vi "RTS MX5 Data.vi"(4 "Measurement Values in":dbl[][](array[numeric]), 6 "Debug":bool, 8 "Error In":errorcluster, 9 "Measurement Date Times":T1(array[cluster]), 10 "Chamber 1 Data in in":T4 {"Room PID Settings"."Room Dehumid Temperature I (*RM Dehum I1)" max=30000 step=1; "Room PID Settings"."Room Dehumid Temperature P (*RM Dehum P1)" max=30000 step=1; "Room PID Settings"."Room Cool Temperature I (*RM Cool I1)" max=30000 step=1; "Room PID Settings"."Room Cool Temperature P (*RM Cool P1)" max=30000 step=1; "Room PID Settings"."Room Heat I (*RM Heat I1)" max=30000 step=1; "Room PID Settings"."Room Heat P (*RM Heat P1)" max=30000 step=1; "Room PID Settings"."Room Humidity I (*RM Hum I1)" max=30000 step=1; "Room PID Settings"."Room Humidity P (*RM Hum P1)" max=30000 step=1; "Room PID Settings"."Room Dry I (*RM Dry I1)" max=30000 step=1; "Room PID Settings"."Room Dry P(*RM Dry P1)" max=30000 step=1; "Station 8"."Voltage (V):Element 1 Avg" format="%.3g"; "Station 8"."Voltage (V):Element 2 Avg" format="%.3g"; "Station 8"."Max Watt Hours" format="%.3g"; "Station 8"."Power Factor:Element 2" format="%.3g"; "Station 8"."Power Factor:Element 1" format="%.3g"; "Station 8"."Apparent Power (VA):Element 2" format="%.3g"; "Station 8"."Apparent Power (VA):Element 1" format="%.3g"; "Station 8"."Frequency (Hz):Element 1" format="%.3g"; "Station 8"."Time:Element 1" format="%.3g"; "Station 8"."Voltage Crest Factor:Element 2" format="%.3g"; "Station 8"."Voltage Crest Factor:Element 1" format="%.3g"; "Station 8"."Voltage Harmonic (%):Element 2" format="%.3g"; "Station 8"."Voltage Harmonic (%):Element 1" format="%.3g"; "Station 8"."Current Crest Factor:Element 2" format="%.3g"; "Station 8"."Current Crest Factor:Element 1" format="%.3g"; "Station 8"."Voltage (V):Element 1" format="%.3g"; "Station 8"."Voltage (V):Element 2" format="%.3g"; "Station 8"."Watt Hours (Wh):Sigma" format="%.3f"; "Station 8"."Power (W):Sigma" format="%.3g"; "Station 8"."Current (A):Element 2" format="%.3g"; "Station 8"."Current (A):Element 1" format="%.3g"; "Station 7"."Voltage (V):Element 1 Avg" format="%.3g"; "Station 7"."Voltage (V):Element 2 Avg" format="%.3g"; "Station 7"."Max Watt Hours" format="%.3g"; "Station 7"."Power Factor:Element 2" format="%.3g"; "Station 7"."Power Factor:Element 1" format="%.3g"; "Station 7"."Apparent Power (VA):Element 2" format="%.3g"; "Station 7"."Apparent Power (VA):Element 1" format="%.3g"; "Station 7"."Frequency (Hz):Element 1" format="%.3g"; "Station 7"."Time:Element 1" format="%.3g"; "Station 7"."Voltage Crest Factor:Element 2" format="%.3g"; "Station 7"."Voltage Crest Factor:Element 1" format="%.3g"; "Station 7"."Voltage Harmonic (%):Element 2" format="%.3g"; "Station 7"."Voltage Harmonic (%):Element 1" format="%.3g"; "Station 7"."Current Crest Factor:Element 2" format="%.3g"; "Station 7"."Current Crest Factor:Element 1" format="%.3g"; "Station 7"."Voltage (V):Element 1" format="%.3g"; "Station 7"."Voltage (V):Element 2" format="%.3g"; "Station 7"."Watt Hours (Wh):Sigma" format="%.3f"; "Station 7"."Power (W):Sigma" format="%.3g"; "Station 7"."Current (A):Element 2" format="%.3g"; "Station 7"."Current (A):Element 1" format="%.3g"; "Station 6"."Voltage (V):Element 1 Avg" format="%.3g"; "Station 6"."Voltage (V):Element 2 Avg" format="%.3g"; "Station 6"."Max Watt Hours" format="%.3g"; "Station 6"."Power Factor:Element 2" format="%.3g"; "Station 6"."Power Factor:Element 1" format="%.3g"; "Station 6"."Apparent Power (VA):Element 2" format="%.3g"; "Station 6"."Apparent Power (VA):Element 1" format="%.3g"; "Station 6"."Frequency (Hz):Element 1" format="%.3g"; "Station 6"."Time:Element 1" format="%.3g"; "Station 6"."Voltage Crest Factor:Element 2" format="%.3g"; "Station 6"."Voltage Crest Factor:Element 1" format="%.3g"; "Station 6"."Voltage Harmonic (%):Element 2" format="%.3g"; "Station 6"."Voltage Harmonic (%):Element 1" format="%.3g"; "Station 6"."Current Crest Factor:Element 2" format="%.3g"; "Station 6"."Current Crest Factor:Element 1" format="%.3g"; "Station 6"."Voltage (V):Element 1" format="%.3g"; "Station 6"."Voltage (V):Element 2" format="%.3g"; "Station 6"."Watt Hours (Wh):Sigma" format="%.3f"; "Station 6"."Power (W):Sigma" format="%.3g"; "Station 6"."Current (A):Element 2" format="%.3g"; "Station 6"."Current (A):Element 1" format="%.3g"; "Station 5"."Voltage (V):Element 1 Avg" format="%.3g"; "Station 5"."Voltage (V):Element 2 Avg" format="%.3g"; "Station 5"."Max Watt Hours" format="%.3g"; "Station 5"."Power Factor:Element 2" format="%.3g"; "Station 5"."Power Factor:Element 1" format="%.3g"; "Station 5"."Apparent Power (VA):Element 2" format="%.3g"; "Station 5"."Apparent Power (VA):Element 1" format="%.3g"; "Station 5"."Frequency (Hz):Element 1" format="%.3g"; "Station 5"."Time:Element 1" format="%.3g"; "Station 5"."Voltage Crest Factor:Element 2" format="%.3g"; "Station 5"."Voltage Crest Factor:Element 1" format="%.3g"; "Station 5"."Voltage Harmonic (%):Element 2" format="%.3g"; "Station 5"."Voltage Harmonic (%):Element 1" format="%.3g"; "Station 5"."Current Crest Factor:Element 2" format="%.3g"; "Station 5"."Current Crest Factor:Element 1" format="%.3g"; "Station 5"."Voltage (V):Element 1" format="%.3g"; "Station 5"."Voltage (V):Element 2" format="%.3g"; "Station 5"."Watt Hours (Wh):Sigma" format="%.3f"; "Station 5"."Power (W):Sigma" format="%.3g"; "Station 5"."Current (A):Element 2" format="%.3g"; "Station 5"."Current (A):Element 1" format="%.3g"; "Station 4"."Voltage (V):Element 1 Avg" format="%.3g"; "Station 4"."Voltage (V):Element 2 Avg" format="%.3g"; "Station 4"."Max Watt Hours" format="%.3g"; "Station 4"."Power Factor:Element 2" format="%.3g"; "Station 4"."Power Factor:Element 1" format="%.3g"; "Station 4"."Apparent Power (VA):Element 2" format="%.3g"; "Station 4"."Apparent Power (VA):Element 1" format="%.3g"; "Station 4"."Frequency (Hz):Element 1" format="%.3g"; "Station 4"."Time:Element 1" format="%.3g"; "Station 4"."Voltage Crest Factor:Element 2" format="%.3g"; "Station 4"."Voltage Crest Factor:Element 1" format="%.3g"; "Station 4"."Voltage Harmonic (%):Element 2" format="%.3g"; "Station 4"."Voltage Harmonic (%):Element 1" format="%.3g"; "Station 4"."Current Crest Factor:Element 2" format="%.3g"; "Station 4"."Current Crest Factor:Element 1" format="%.3g"; "Station 4"."Voltage (V):Element 1" format="%.3g"; "Station 4"."Voltage (V):Element 2" format="%.3g"; "Station 4"."Watt Hours (Wh):Sigma" format="%.3f"; "Station 4"."Power (W):Sigma" format="%.3g"; "Station 4"."Current (A):Element 2" format="%.3g"; "Station 4"."Current (A):Element 1" format="%.3g"; "Station 3"."Voltage (V):Element 1 Avg" format="%.3g"; "Station 3"."Voltage (V):Element 2 Avg" format="%.3g"; "Station 3"."Max Watt Hours" format="%.3g"; "Station 3"."Power Factor:Element 2" format="%.3g"; "Station 3"."Power Factor:Element 1" format="%.3g"; "Station 3"."Apparent Power (VA):Element 2" format="%.3g"; "Station 3"."Apparent Power (VA):Element 1" format="%.3g"; "Station 3"."Frequency (Hz):Element 1" format="%.3g"; "Station 3"."Time:Element 1" format="%.3g"; "Station 3"."Voltage Crest Factor:Element 2" format="%.3g"; "Station 3"."Voltage Crest Factor:Element 1" format="%.3g"; "Station 3"."Voltage Harmonic (%):Element 2" format="%.3g"; "Station 3"."Voltage Harmonic (%):Element 1" format="%.3g"; "Station 3"."Current Crest Factor:Element 2" format="%.3g"; "Station 3"."Current Crest Factor:Element 1" format="%.3g"; "Station 3"."Voltage (V):Element 1" format="%.3g"; "Station 3"."Voltage (V):Element 2" format="%.3g"; "Station 3"."Watt Hours (Wh):Sigma" format="%.3f"; "Station 3"."Power (W):Sigma" format="%.3g"; "Station 3"."Current (A):Element 2" format="%.3g"; "Station 3"."Current (A):Element 1" format="%.3g"; "Station 2"."Voltage (V):Element 1 Avg" format="%.3g"; "Station 2"."Voltage (V):Element 2 Avg" format="%.3g"; "Station 2"."Max Watt Hours" format="%.3g"; "Station 2"."Power Factor:Element 2" format="%.3g"; "Station 2"."Power Factor:Element 1" format="%.3g"; "Station 2"."Apparent Power (VA):Element 2" format="%.3g"; "Station 2"."Apparent Power (VA):Element 1" format="%.3g"; "Station 2"."Frequency (Hz):Element 1" format="%.3g"; "Station 2"."Time:Element 1" format="%.3g"; "Station 2"."Voltage Crest Factor:Element 2" format="%.3g"; "Station 2"."Voltage Crest Factor:Element 1" format="%.3g"; "Station 2"."Voltage Harmonic (%):Element 2" format="%.3g"; "Station 2"."Voltage Harmonic (%):Element 1" format="%.3g"; "Station 2"."Current Crest Factor:Element 2" format="%.3g"; "Station 2"."Current Crest Factor:Element 1" format="%.3g"; "Station 2"."Voltage (V):Element 1" format="%.3g"; "Station 2"."Voltage (V):Element 2" format="%.3g"; "Station 2"."Watt Hours (Wh):Sigma" format="%.3f"; "Station 2"."Power (W):Sigma" format="%.3g"; "Station 2"."Current (A):Element 2" format="%.3g"; "Station 2"."Current (A):Element 1" format="%.3g"; "Station 1"."Voltage (V):Element 1 Avg" format="%.3g"; "Station 1"."Voltage (V):Element 2 Avg" format="%.3g"; "Station 1"."Max Watt Hours" format="%.3g"; "Station 1"."Power Factor:Element 2" format="%.3g"; "Station 1"."Power Factor:Element 1" format="%.3g"; "Station 1"."Apparent Power (VA):Element 2" format="%.3g"; "Station 1"."Apparent Power (VA):Element 1" format="%.3g"; "Station 1"."Frequency (Hz):Element 1" format="%.3g"; "Station 1"."Time:Element 1" format="%.3g"; "Station 1"."Voltage Crest Factor:Element 2" format="%.3g"; "Station 1"."Voltage Crest Factor:Element 1" format="%.3g"; "Station 1"."Voltage Harmonic (%):Element 2" format="%.3g"; "Station 1"."Voltage Harmonic (%):Element 1" format="%.3g"; "Station 1"."Current Crest Factor:Element 2" format="%.3g"; "Station 1"."Current Crest Factor:Element 1" format="%.3g"; "Station 1"."Voltage (V):Element 1" format="%.3g"; "Station 1"."Voltage (V):Element 2" format="%.3g"; "Station 1"."Watt Hours (Wh):Sigma" format="%.3f"; "Station 1"."Power (W):Sigma" format="%.3g"; "Station 1"."Current (A):Element 2" format="%.3g"; "Station 1"."Current (A):Element 1" format="%.3g"}, 11 "MX":T2={"Base Time"=0, "Session Number"=0, "Last Data Number"={"High"=-1, "Low"=4294967295}, "Channel List"=[], "FIFO Number (0)"=0, "Channel Number (1)"=1, "Select FIFO or Channel (F:Channel)"=FALSE, "MX100 Data"={"Measurement Values out"=[], "Date/Time"=""}} {"Channel Number (1)" min=1 max=60 step=1; "FIFO Number (0)" min=-1 max=2 step=1}) -> (0 "Error Out":errorcluster, 2 "Chamber 1 Data out":T4 {"Room PID Settings"."Room Dehumid Temperature I (*RM Dehum I1)" max=30000 step=1; "Room PID Settings"."Room Dehumid Temperature P (*RM Dehum P1)" max=30000 step=1; "Room PID Settings"."Room Cool Temperature I (*RM Cool I1)" max=30000 step=1; "Room PID Settings"."Room Cool Temperature P (*RM Cool P1)" max=30000 step=1; "Room PID Settings"."Room Heat I (*RM Heat I1)" max=30000 step=1; "Room PID Settings"."Room Heat P (*RM Heat P1)" max=30000 step=1; "Room PID Settings"."Room Humidity I (*RM Hum I1)" max=30000 step=1; "Room PID Settings"."Room Humidity P (*RM Hum P1)" max=30000 step=1; "Room PID Settings"."Room Dry I (*RM Dry I1)" max=30000 step=1; "Room PID Settings"."Room Dry P(*RM Dry P1)" max=30000 step=1; "Station 8"."Voltage (V):Element 1 Avg" format="%.3g"; "Station 8"."Voltage (V):Element 2 Avg" format="%.3g"; "Station 8"."Max Watt Hours" format="%.3g"; "Station 8"."Power Factor:Element 2" format="%.3g"; "Station 8"."Power Factor:Element 1" format="%.3g"; "Station 8"."Apparent Power (VA):Element 2" format="%.3g"; "Station 8"."Apparent Power (VA):Element 1" format="%.3g"; "Station 8"."Frequency (Hz):Element 1" format="%.3g"; "Station 8"."Time:Element 1" format="%.3g"; "Station 8"."Voltage Crest Factor:Element 2" format="%.3g"; "Station 8"."Voltage Crest Factor:Element 1" format="%.3g"; "Station 8"."Voltage Harmonic (%):Element 2" format="%.3g"; "Station 8"."Voltage Harmonic (%):Element 1" format="%.3g"; "Station 8"."Current Crest Factor:Element 2" format="%.3g"; "Station 8"."Current Crest Factor:Element 1" format="%.3g"; "Station 8"."Voltage (V):Element 1" format="%.3g"; "Station 8"."Voltage (V):Element 2" format="%.3g"; "Station 8"."Watt Hours (Wh):Sigma" format="%.3f"; "Station 8"."Power (W):Sigma" format="%.3g"; "Station 8"."Current (A):Element 2" format="%.3g"; "Station 8"."Current (A):Element 1" format="%.3g"; "Station 7"."Voltage (V):Element 1 Avg" format="%.3g"; "Station 7"."Voltage (V):Element 2 Avg" format="%.3g"; "Station 7"."Max Watt Hours" format="%.3g"; "Station 7"."Power Factor:Element 2" format="%.3g"; "Station 7"."Power Factor:Element 1" format="%.3g"; "Station 7"."Apparent Power (VA):Element 2" format="%.3g"; "Station 7"."Apparent Power (VA):Element 1" format="%.3g"; "Station 7"."Frequency (Hz):Element 1" format="%.3g"; "Station 7"."Time:Element 1" format="%.3g"; "Station 7"."Voltage Crest Factor:Element 2" format="%.3g"; "Station 7"."Voltage Crest Factor:Element 1" format="%.3g"; "Station 7"."Voltage Harmonic (%):Element 2" format="%.3g"; "Station 7"."Voltage Harmonic (%):Element 1" format="%.3g"; "Station 7"."Current Crest Factor:Element 2" format="%.3g"; "Station 7"."Current Crest Factor:Element 1" format="%.3g"; "Station 7"."Voltage (V):Element 1" format="%.3g"; "Station 7"."Voltage (V):Element 2" format="%.3g"; "Station 7"."Watt Hours (Wh):Sigma" format="%.3f"; "Station 7"."Power (W):Sigma" format="%.3g"; "Station 7"."Current (A):Element 2" format="%.3g"; "Station 7"."Current (A):Element 1" format="%.3g"; "Station 6"."Voltage (V):Element 1 Avg" format="%.3g"; "Station 6"."Voltage (V):Element 2 Avg" format="%.3g"; "Station 6"."Max Watt Hours" format="%.3g"; "Station 6"."Power Factor:Element 2" format="%.3g"; "Station 6"."Power Factor:Element 1" format="%.3g"; "Station 6"."Apparent Power (VA):Element 2" format="%.3g"; "Station 6"."Apparent Power (VA):Element 1" format="%.3g"; "Station 6"."Frequency (Hz):Element 1" format="%.3g"; "Station 6"."Time:Element 1" format="%.3g"; "Station 6"."Voltage Crest Factor:Element 2" format="%.3g"; "Station 6"."Voltage Crest Factor:Element 1" format="%.3g"; "Station 6"."Voltage Harmonic (%):Element 2" format="%.3g"; "Station 6"."Voltage Harmonic (%):Element 1" format="%.3g"; "Station 6"."Current Crest Factor:Element 2" format="%.3g"; "Station 6"."Current Crest Factor:Element 1" format="%.3g"; "Station 6"."Voltage (V):Element 1" format="%.3g"; "Station 6"."Voltage (V):Element 2" format="%.3g"; "Station 6"."Watt Hours (Wh):Sigma" format="%.3f"; "Station 6"."Power (W):Sigma" format="%.3g"; "Station 6"."Current (A):Element 2" format="%.3g"; "Station 6"."Current (A):Element 1" format="%.3g"; "Station 5"."Voltage (V):Element 1 Avg" format="%.3g"; "Station 5"."Voltage (V):Element 2 Avg" format="%.3g"; "Station 5"."Max Watt Hours" format="%.3g"; "Station 5"."Power Factor:Element 2" format="%.3g"; "Station 5"."Power Factor:Element 1" format="%.3g"; "Station 5"."Apparent Power (VA):Element 2" format="%.3g"; "Station 5"."Apparent Power (VA):Element 1" format="%.3g"; "Station 5"."Frequency (Hz):Element 1" format="%.3g"; "Station 5"."Time:Element 1" format="%.3g"; "Station 5"."Voltage Crest Factor:Element 2" format="%.3g"; "Station 5"."Voltage Crest Factor:Element 1" format="%.3g"; "Station 5"."Voltage Harmonic (%):Element 2" format="%.3g"; "Station 5"."Voltage Harmonic (%):Element 1" format="%.3g"; "Station 5"."Current Crest Factor:Element 2" format="%.3g"; "Station 5"."Current Crest Factor:Element 1" format="%.3g"; "Station 5"."Voltage (V):Element 1" format="%.3g"; "Station 5"."Voltage (V):Element 2" format="%.3g"; "Station 5"."Watt Hours (Wh):Sigma" format="%.3f"; "Station 5"."Power (W):Sigma" format="%.3g"; "Station 5"."Current (A):Element 2" format="%.3g"; "Station 5"."Current (A):Element 1" format="%.3g"; "Station 4"."Voltage (V):Element 1 Avg" format="%.3g"; "Station 4"."Voltage (V):Element 2 Avg" format="%.3g"; "Station 4"."Max Watt Hours" format="%.3g"; "Station 4"."Power Factor:Element 2" format="%.3g"; "Station 4"."Power Factor:Element 1" format="%.3g"; "Station 4"."Apparent Power (VA):Element 2" format="%.3g"; "Station 4"."Apparent Power (VA):Element 1" format="%.3g"; "Station 4"."Frequency (Hz):Element 1" format="%.3g"; "Station 4"."Time:Element 1" format="%.3g"; "Station 4"."Voltage Crest Factor:Element 2" format="%.3g"; "Station 4"."Voltage Crest Factor:Element 1" format="%.3g"; "Station 4"."Voltage Harmonic (%):Element 2" format="%.3g"; "Station 4"."Voltage Harmonic (%):Element 1" format="%.3g"; "Station 4"."Current Crest Factor:Element 2" format="%.3g"; "Station 4"."Current Crest Factor:Element 1" format="%.3g"; "Station 4"."Voltage (V):Element 1" format="%.3g"; "Station 4"."Voltage (V):Element 2" format="%.3g"; "Station 4"."Watt Hours (Wh):Sigma" format="%.3f"; "Station 4"."Power (W):Sigma" format="%.3g"; "Station 4"."Current (A):Element 2" format="%.3g"; "Station 4"."Current (A):Element 1" format="%.3g"; "Station 3"."Voltage (V):Element 1 Avg" format="%.3g"; "Station 3"."Voltage (V):Element 2 Avg" format="%.3g"; "Station 3"."Max Watt Hours" format="%.3g"; "Station 3"."Power Factor:Element 2" format="%.3g"; "Station 3"."Power Factor:Element 1" format="%.3g"; "Station 3"."Apparent Power (VA):Element 2" format="%.3g"; "Station 3"."Apparent Power (VA):Element 1" format="%.3g"; "Station 3"."Frequency (Hz):Element 1" format="%.3g"; "Station 3"."Time:Element 1" format="%.3g"; "Station 3"."Voltage Crest Factor:Element 2" format="%.3g"; "Station 3"."Voltage Crest Factor:Element 1" format="%.3g"; "Station 3"."Voltage Harmonic (%):Element 2" format="%.3g"; "Station 3"."Voltage Harmonic (%):Element 1" format="%.3g"; "Station 3"."Current Crest Factor:Element 2" format="%.3g"; "Station 3"."Current Crest Factor:Element 1" format="%.3g"; "Station 3"."Voltage (V):Element 1" format="%.3g"; "Station 3"."Voltage (V):Element 2" format="%.3g"; "Station 3"."Watt Hours (Wh):Sigma" format="%.3f"; "Station 3"."Power (W):Sigma" format="%.3g"; "Station 3"."Current (A):Element 2" format="%.3g"; "Station 3"."Current (A):Element 1" format="%.3g"; "Station 2"."Voltage (V):Element 1 Avg" format="%.3g"; "Station 2"."Voltage (V):Element 2 Avg" format="%.3g"; "Station 2"."Max Watt Hours" format="%.3g"; "Station 2"."Power Factor:Element 2" format="%.3g"; "Station 2"."Power Factor:Element 1" format="%.3g"; "Station 2"."Apparent Power (VA):Element 2" format="%.3g"; "Station 2"."Apparent Power (VA):Element 1" format="%.3g"; "Station 2"."Frequency (Hz):Element 1" format="%.3g"; "Station 2"."Time:Element 1" format="%.3g"; "Station 2"."Voltage Crest Factor:Element 2" format="%.3g"; "Station 2"."Voltage Crest Factor:Element 1" format="%.3g"; "Station 2"."Voltage Harmonic (%):Element 2" format="%.3g"; "Station 2"."Voltage Harmonic (%):Element 1" format="%.3g"; "Station 2"."Current Crest Factor:Element 2" format="%.3g"; "Station 2"."Current Crest Factor:Element 1" format="%.3g"; "Station 2"."Voltage (V):Element 1" format="%.3g"; "Station 2"."Voltage (V):Element 2" format="%.3g"; "Station 2"."Watt Hours (Wh):Sigma" format="%.3f"; "Station 2"."Power (W):Sigma" format="%.3g"; "Station 2"."Current (A):Element 2" format="%.3g"; "Station 2"."Current (A):Element 1" format="%.3g"; "Station 1"."Voltage (V):Element 1 Avg" format="%.3g"; "Station 1"."Voltage (V):Element 2 Avg" format="%.3g"; "Station 1"."Max Watt Hours" format="%.3g"; "Station 1"."Power Factor:Element 2" format="%.3g"; "Station 1"."Power Factor:Element 1" format="%.3g"; "Station 1"."Apparent Power (VA):Element 2" format="%.3g"; "Station 1"."Apparent Power (VA):Element 1" format="%.3g"; "Station 1"."Frequency (Hz):Element 1" format="%.3g"; "Station 1"."Time:Element 1" format="%.3g"; "Station 1"."Voltage Crest Factor:Element 2" format="%.3g"; "Station 1"."Voltage Crest Factor:Element 1" format="%.3g"; "Station 1"."Voltage Harmonic (%):Element 2" format="%.3g"; "Station 1"."Voltage Harmonic (%):Element 1" format="%.3g"; "Station 1"."Current Crest Factor:Element 2" format="%.3g"; "Station 1"."Current Crest Factor:Element 1" format="%.3g"; "Station 1"."Voltage (V):Element 1" format="%.3g"; "Station 1"."Voltage (V):Element 2" format="%.3g"; "Station 1"."Watt Hours (Wh):Sigma" format="%.3f"; "Station 1"."Power (W):Sigma" format="%.3g"; "Station 1"."Current (A):Element 2" format="%.3g"; "Station 1"."Current (A):Element 1" format="%.3g"})   [LabVIEW 2016]
uses:
  Type Definitions/RTS Chamber Data.ctl
  Utility/Type Definitions/UTILITY Power Data.ctl
  Type Definitions/RTS Chamber TCs.ctl
  Type Definitions/RTS MX5 AUX Data.ctl
  Drivers/WAGO 750-881/Type Definitions/Wago Door Relays.ctl
  Drivers/WAGO 750-881/Type Definitions/Wago Contactor Settings.ctl
  Drivers/WAGO 750-881/Type Definitions/Wago Ground Leakage.ctl
  Drivers/WAGO 750-881/Type Definitions/Wago Measured Input Data.ctl
  Drivers/WAGO 750-881/Type Definitions/Wago Room Setpoint Targets.ctl
  Drivers/WAGO 750-881/Type Definitions/Wago Room PID Settings.ctl
  Drivers/WAGO 750-881/Type Definitions/Wago Room Condtions.ctl
  Drivers/Yokogawa MX100/Type Definitions/MX100 Initialization.ctl
  Drivers/Yokogawa MX100/Type Definitions/MX100 Data.ctl
panel:
  # "APLUS"
  # "MX100"
  # "Wago Controller"
  # "APLUS"
  # "MX100"
  # "Wago Controller"
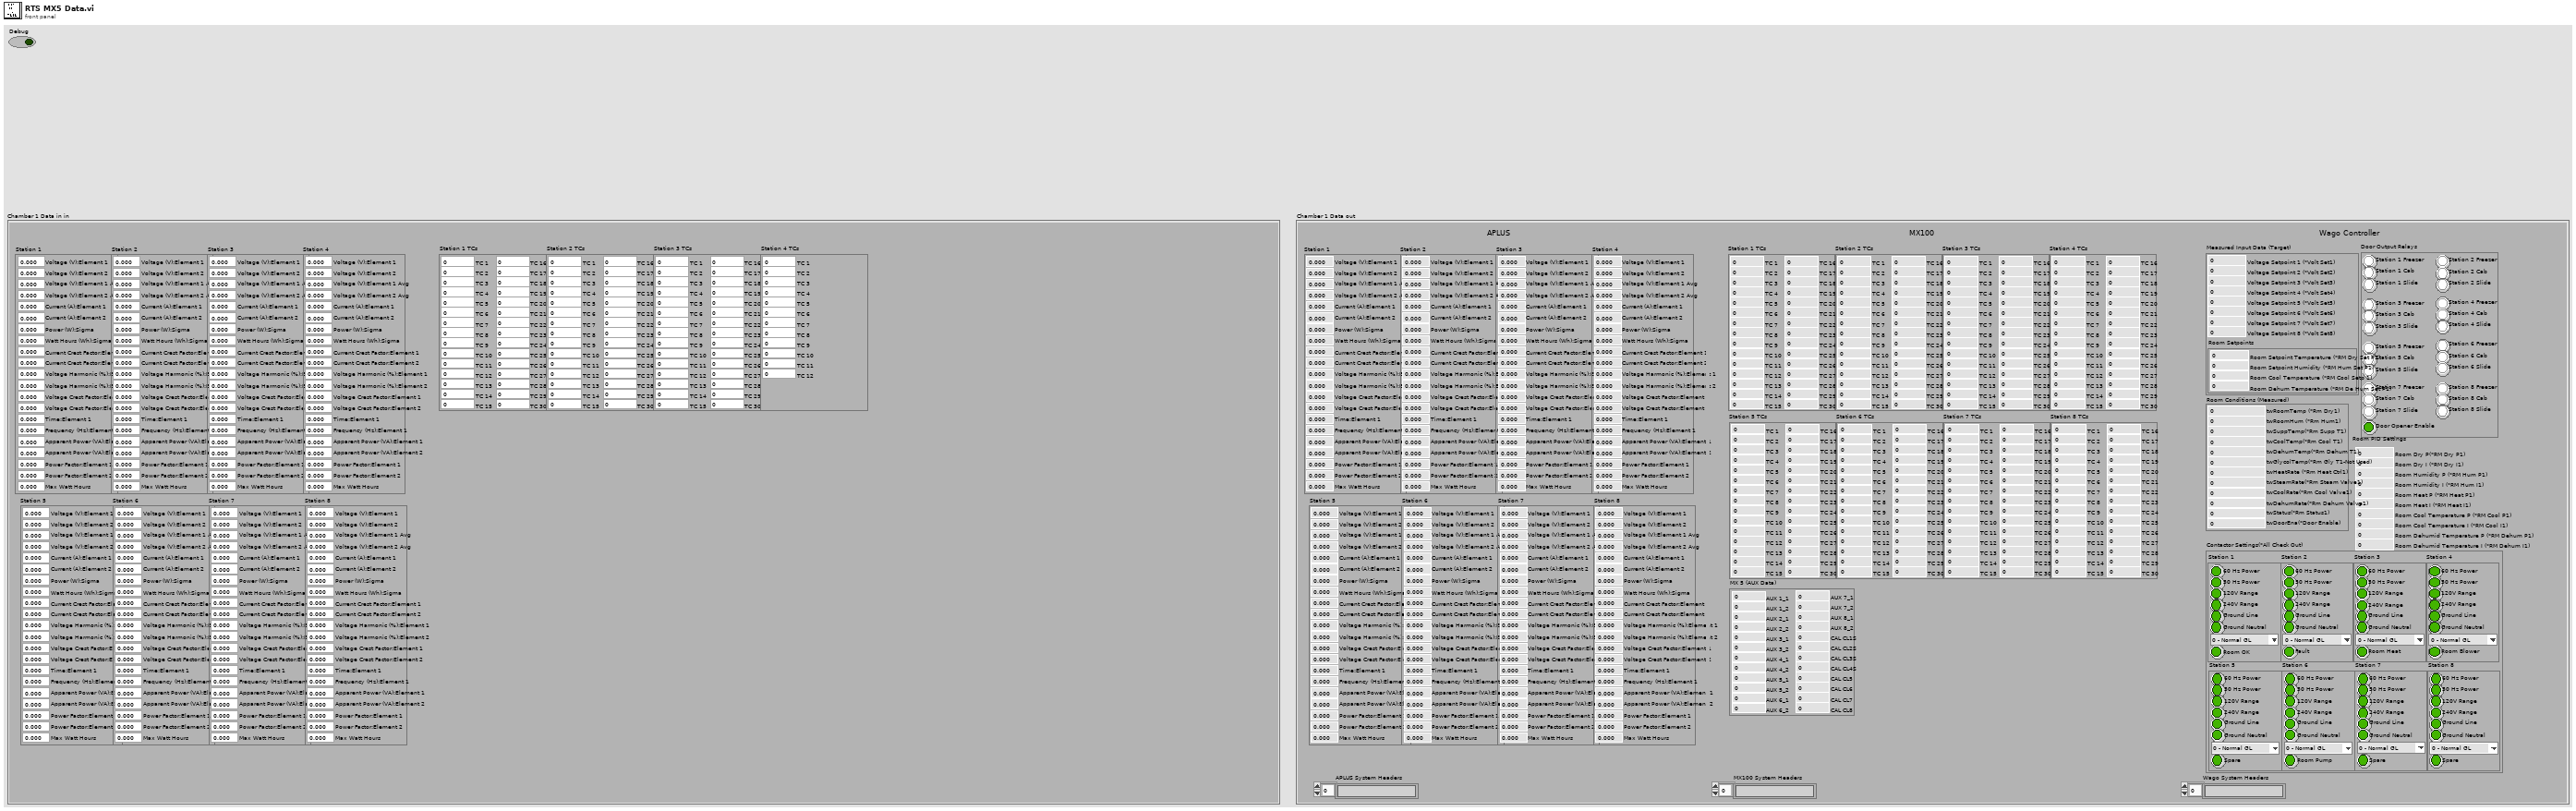
[diagram p1: front panel]
types:
  T1 = cluster{"Measurement Time":u32, "Milli Second":i32}[]
  T2 = typedef "MX100 Initialization.ctl" = cluster{"Base Time":i32, "Session Number":i32, "Last Data Number":cluster{"High":i32, "Low":u32}, "Channel List":string[], "FIFO Number (0)":i32, "Channel Number (1)":i32, "Select FIFO or Channel (F:Channel)":bool, "MX100 Data":T3}
  T3 = typedef "MX100 Data.ctl" = cluster{"Measurement Values out":dbl[], "Date/Time":string}
  T4 = typedef "RTS Chamber Data.ctl" = cluster{"Station 1":T5, "Station 2":T5, "Station 3":T5, "Station 4":T5, "Station 5":T5, "Station 6":T5, "Station 7":T5, "Station 8":T5, "Station 1 TCs":T6, "Station 2 TCs":T6, "Station 3 TCs":T6, "Station 4 TCs":T6, "Station 5 TCs":T6, "Station 6 TCs":T6, "Station 7 TCs":T6, "Station 8 TCs":T6, "MX 5 (AUX Data)":T7, "Door Output Relays":T8, "Contactor Settings(*All Check Out)":T9, "Measured Input Data (Target)":T11, "Room PID Settings":T13, "Room Conditions (Measured)":T14, "APLUS System Headers":string[], "MX100 System Headers":string[], "Wago System Headers":string[]}
  T5 = typedef "UTILITY Power Data.ctl" = cluster{"Current (A):Element 1":dbl, "Current (A):Element 2":dbl, "Power (W):Sigma":dbl, "Watt Hours (Wh):Sigma":dbl, "Voltage (V):Element 2":dbl, "Voltage (V):Element 1":dbl, "Current Crest Factor:Element 1":dbl, "Current Crest Factor:Element 2":dbl, "Voltage Harmonic (%):Element 1":dbl, "Voltage Harmonic (%):Element 2":dbl, "Voltage Crest Factor:Element 1":dbl, "Voltage Crest Factor:Element 2":dbl, "Time:Element 1":dbl, "Frequency (Hz):Element 1":dbl, "Apparent Power (VA):Element 1":dbl, "Apparent Power (VA):Element 2":dbl, "Power Factor:Element 1":dbl, "Power Factor:Element 2":dbl, "Max Watt Hours":dbl, "Voltage (V):Element 2 Avg":dbl, "Voltage (V):Element 1 Avg":dbl}
  T6 = typedef "RTS Chamber TCs.ctl" = cluster{"TC 1":dbl, "TC 2":dbl, "TC 3":dbl, "TC 4":dbl, "TC 5":dbl, "TC 6":dbl, "TC 7":dbl, "TC 8":dbl, "TC 9":dbl, "TC 10":dbl, "TC 11":dbl, "TC 12":dbl, "TC 13":dbl, "TC 14":dbl, "TC 15":dbl, "TC 16":dbl, "TC 17":dbl, "TC 18":dbl, "TC 19":dbl, "TC 20":dbl, "TC 21":dbl, "TC 22":dbl, "TC 23":dbl, "TC 24":dbl, "TC 25":dbl, "TC 26":dbl, "TC 27":dbl, "TC 28":dbl, "TC 29":dbl, "TC 30":dbl}
  T7 = typedef "RTS MX5 AUX Data.ctl" = cluster{"AUX 1_1":dbl, "AUX 1_2":dbl, "AUX 2_1":dbl, "AUX 2_2":dbl, "AUX 3_1":dbl, "AUX 3_2":dbl, "AUX 4_1":dbl, "AUX 4_2":dbl, "AUX 5_1":dbl, "AUX 5_2":dbl, "AUX 6_1":dbl, "AUX 6_2":dbl, "AUX 7_1":dbl, "AUX 7_2":dbl, "AUX 8_1":dbl, "AUX 8_2":dbl, "CAL CL1S":dbl, "CAL CL2S":dbl, "CAL CL3S":dbl, "CAL CL4S":dbl, "CAL CL5":dbl, "CAL CL6":dbl, "CAL CL7":dbl, "CAL CL8":dbl}
  T8 = typedef "Wago Door Relays.ctl" = cluster{"Station 1 Freezer":bool, "Station 1 Cab":bool, "Station 1 Slide":bool, "Station 2 Freezer":bool, "Station 2 Cab":bool, "Station 2 Slide":bool, "Station 3 Freezer":bool, "Station 3 Cab":bool, "Station 3 Slide":bool, "Station 4 Freezer":bool, "Station 4 Cab":bool, "Station 4 Slide":bool, "Station 5 Freezer":bool, "Station 5 Cab":bool, "Station 5 Slide":bool, "Station 6 Freezer":bool, "Station 6 Cab":bool, "Station 6 Slide":bool, "Station 7 Freezer":bool, "Station 7 Cab":bool, "Station 7 Slide":bool, "Station 8 Freezer":bool, "Station 8 Cab":bool, "Station 8 Slide":bool, "Door Opener Enable":bool}
  T9 = typedef "Wago Contactor Settings.ctl" = cluster{"Station 1":cluster{"60 Hz Power":bool, "50 Hz Power":bool, "120V Range":bool, "240V Range":bool, "Ground Line":bool, "Ground Neutral":bool, "Room OK":bool, "Ground Leakage":T10}, "Station 2":cluster{"60 Hz Power":bool, "50 Hz Power":bool, "120V Range":bool, "240V Range":bool, "Ground Line":bool, "Ground Neutral":bool, "Fault":bool, "Ground Leakage":T10}, "Station 3":cluster{"60 Hz Power":bool, "50 Hz Power":bool, "120V Range":bool, "240V Range":bool, "Ground Line":bool, "Ground Neutral":bool, "Room Heat":bool, "Ground Leakage":T10}, "Station 4":cluster{"60 Hz Power":bool, "50 Hz Power":bool, "120V Range":bool, "240V Range":bool, "Ground Line":bool, "Ground Neutral":bool, "Room Blower":bool, "Ground Leakage":T10}, "Station 5":cluster{"60 Hz Power":bool, "50 Hz Power":bool, "120V Range":bool, "240V Range":bool, "Ground Line":bool, "Ground Neutral":bool, "Spare":bool, "Ground Leakage":T10}, "Station 6":cluster{"60 Hz Power":bool, "50 Hz Power":bool, "120V Range":bool, "240V Range":bool, "Ground Line":bool, "Ground Neutral":bool, "Room Pump":bool, "Ground Leakage":T10}, "Station 7":cluster{"60 Hz Power":bool, "50 Hz Power":bool, "120V Range":bool, "240V Range":bool, "Ground Line":bool, "Ground Neutral":bool, "Spare":bool, "Ground Leakage":T10}, "Station 8":cluster{"60 Hz Power":bool, "50 Hz Power":bool, "120V Range":bool, "240V Range":bool, "Ground Line":bool, "Ground Neutral":bool, "Spare":bool, "Ground Leakage":T10}}
  T10 = typedef "Wago Ground Leakage.ctl" = enum16{"0 - Normal GL", "1 - Measure GL"}
  T11 = typedef "Wago Measured Input Data.ctl" = cluster{"Voltage Setpoint 1 (*Volt Set1)":dbl, "Voltage Setpoint 2 (*Volt Set2)":dbl, "Voltage Setpoint 3 (*Volt Set3)":dbl, "Voltage Setpoint 4 (*Volt Set4)":dbl, "Voltage Setpoint 5 (*Volt Set5)":dbl, "Voltage Setpoint 6 (*Volt Set6)":dbl, "Voltage Setpoint 7 (*Volt Set7)":dbl, "Voltage Setpoint 8 (*Volt Set8)":dbl, "Room Setpoints":T12}
  T12 = typedef "Wago Room Setpoint Targets.ctl" = cluster{"Room Setpoint Temperature (*RM Dry Set P1)":dbl, "Room Setpoint Humidity (*RM Hum Set P1)":dbl, "Room Cool Temperature (*RM Cool Setp 1)":dbl, "Room Dehum Temperature (*RM De Hum Set P1)":dbl}
  T13 = typedef "Wago Room PID Settings.ctl" = cluster{"Room Dry P(*RM Dry P1)":u16, "Room Dry I (*RM Dry I1)":u16, "Room Humidity P (*RM Hum P1)":u16, "Room Humidity I (*RM Hum I1)":u16, "Room Heat P (*RM Heat P1)":u16, "Room Heat I (*RM Heat I1)":u16, "Room Cool Temperature P (*RM Cool P1)":u16, "Room Cool Temperature I (*RM Cool I1)":u16, "Room Dehumid Temperature P (*RM Dehum P1)":u16, "Room Dehumid Temperature I (*RM Dehum I1)":u16}
  T14 = typedef "Wago Room Condtions.ctl" = cluster{"twDoorEna(*Door Enable)":u16, "twStatus(*Rm Status1)":u16, "twRoomTemp (*Rm Dry1)":dbl, "twRoomHum (*Rm Hum1)":dbl, "twSuppTemp(*Rm Supp T1)":dbl, "twCoolTemp(*Rm Cool T1)":dbl, "twDehumTemp(*Rm Dehum T1)":dbl, "twGlycolTemp(*Rm Gly T1-Not Used)":dbl, "twDehumRate(*Rm Dehum Valve1)":dbl, "twCoolRate(*Rm Cool Valve1)":dbl, "twSteamRate(*Rm Steam Valve1)":dbl, "twHeatRate (*Rm Heat Ctrl1)":dbl}
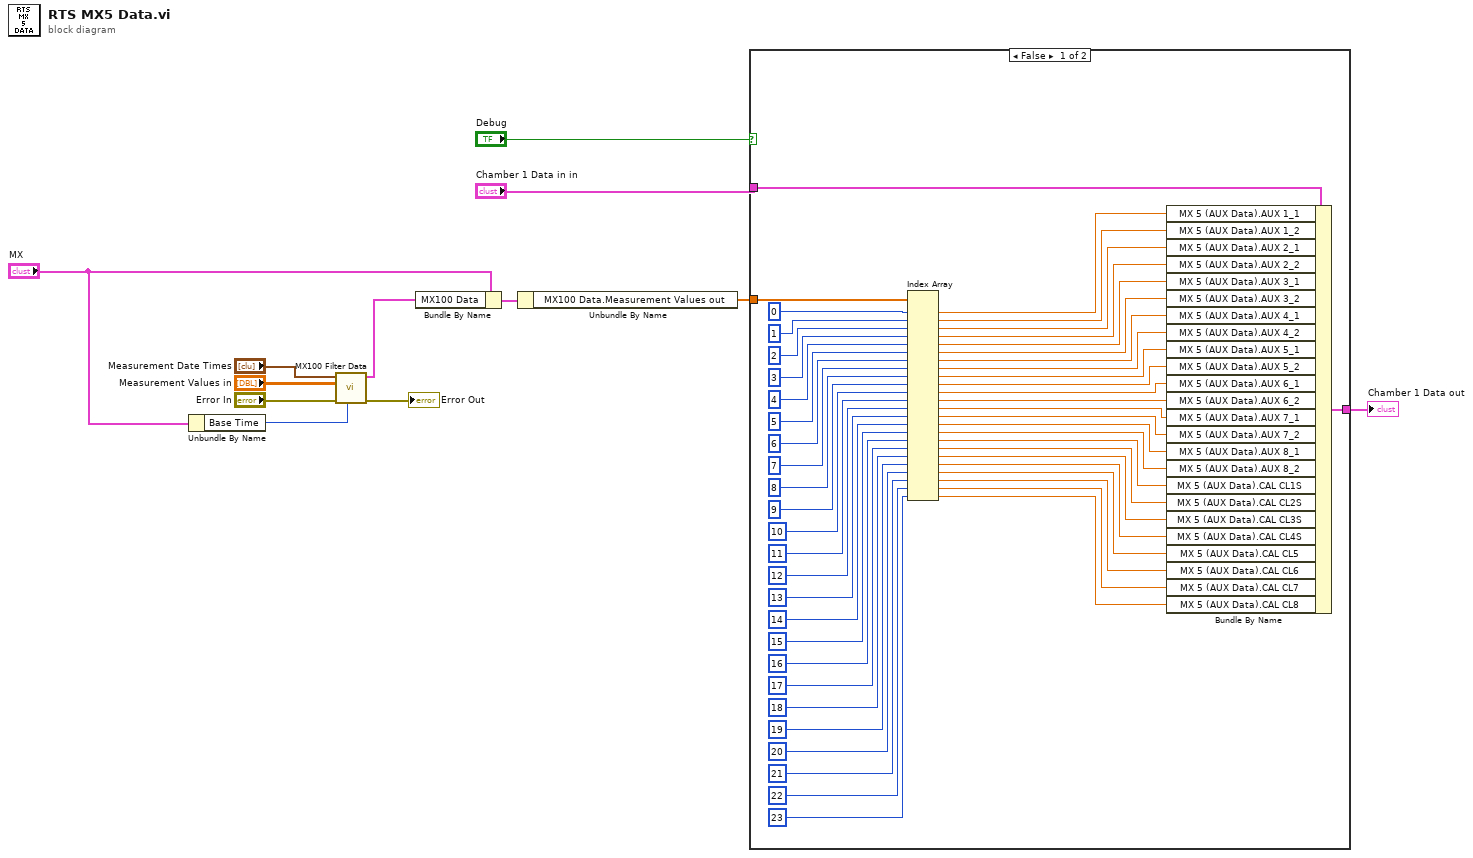
[diagram p0: block diagram]
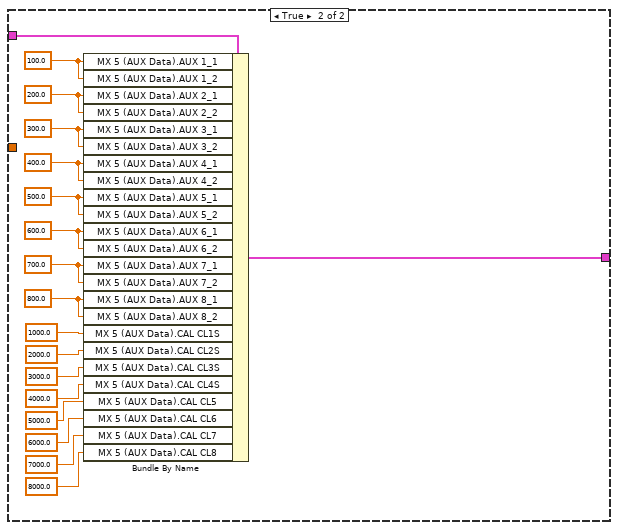
[diagram p2: hidden frame]
diagram:
  n1 = Unbundle By Name("MX") -> ("Base Time"=w8:i32)
  n2 = call "MX100 Filter Data.vi"("Base Time"=w8, "error in (no error)"="Error In", "Measurement Values in"="Measurement Values in", "Measurement Date Times"="Measurement Date Times") -> ("error out"=→"Error Out":errorcluster, "MX100 Data"=w7:T3)  [unwired: 6 in]
  n3 = Bundle By Name(cluster="MX", "MX100 Data"=w7) -> (w3:T2)
  n4 = Unbundle By Name(w3) -> ("MX100 Data.Measurement Values out"=w9:dbl[])
  n5 = case shown="False" "Debug" {
    tunnel: "Chamber 1 Data in in" -> [w39 w81]
    tunnel: [w38 w80] -> w11
    tunnel: w9 -> [w37 _]
    frame False {
      n6 = Index Array(array=w37, index #1=0 ("index"), index #2=1 ("index"), index #3=2 ("index"), index #4=3 ("index"), index #5=4 ("index"), index #6=5 ("index"), index #7=6 ("index"), index #8=7 ("index"), index #9=8 ("index"), index #10=9 ("index"), index #11=10 ("index"), index #12=11 ("index"), index #13=12 ("index"), index #14=13 ("index"), index #15=14 ("index"), index #16=15 ("index"), index #17=16 ("index"), index #18=17 ("index"), index #19=18 ("index"), index #20=19 ("index"), index #21=20 ("index"), index #22=21 ("index"), index #23=22 ("index"), index #24=23 ("index")) -> (element #1=w36:dbl, element #2=w35:dbl, element #3=w34:dbl, element #4=w33:dbl, element #5=w32:dbl, element #6=w31:dbl, element #7=w30:dbl, element #8=w29:dbl, element #9=w28:dbl, element #10=w27:dbl, element #11=w26:dbl, element #12=w25:dbl, element #13=w24:dbl, element #14=w23:dbl, element #15=w22:dbl, element #16=w21:dbl, element #17=w20:dbl, element #18=w19:dbl, element #19=w18:dbl, element #20=w17:dbl, element #21=w16:dbl, element #22=w15:dbl, element #23=w14:dbl, element #24=w13:dbl)
      n7 = Bundle By Name(cluster=w39, "MX 5 (AUX Data).AUX 1_1"=w36, "MX 5 (AUX Data).AUX 1_2"=w35, "MX 5 (AUX Data).AUX 2_1"=w34, "MX 5 (AUX Data).AUX 2_2"=w33, "MX 5 (AUX Data).AUX 3_1"=w32, "MX 5 (AUX Data).AUX 3_2"=w31, "MX 5 (AUX Data).AUX 4_1"=w30, "MX 5 (AUX Data).AUX 4_2"=w29, "MX 5 (AUX Data).AUX 5_1"=w28, "MX 5 (AUX Data).AUX 5_2"=w27, "MX 5 (AUX Data).AUX 6_1"=w26, "MX 5 (AUX Data).AUX 6_2"=w25, "MX 5 (AUX Data).AUX 7_1"=w24, "MX 5 (AUX Data).AUX 7_2"=w23, "MX 5 (AUX Data).AUX 8_1"=w22, "MX 5 (AUX Data).AUX 8_2"=w21, "MX 5 (AUX Data).CAL CL1S"=w20, "MX 5 (AUX Data).CAL CL2S"=w19, "MX 5 (AUX Data).CAL CL3S"=w18, "MX 5 (AUX Data).CAL CL4S"=w17, "MX 5 (AUX Data).CAL CL5"=w16, "MX 5 (AUX Data).CAL CL6"=w15, "MX 5 (AUX Data).CAL CL7"=w14, "MX 5 (AUX Data).CAL CL8"=w13) -> (w38:T4)
    }
    frame True {
      w72 = 800.0 ("MX 5 (AUX Data).AUX 2_1")
      w73 = 700.0 ("MX 5 (AUX Data).AUX 2_1")
      w74 = 600.0 ("MX 5 (AUX Data).AUX 2_1")
      w75 = 500.0 ("MX 5 (AUX Data).AUX 2_1")
      w76 = 400.0 ("MX 5 (AUX Data).AUX 2_1")
      w77 = 300.0 ("MX 5 (AUX Data).AUX 2_1")
      w78 = 200.0 ("MX 5 (AUX Data).AUX 2_1")
      w79 = 100.0 ("MX 5 (AUX Data).AUX 1_1")
      n8 = Bundle By Name(cluster=w81, "MX 5 (AUX Data).AUX 1_1"=w79, "MX 5 (AUX Data).AUX 1_2"=w79, "MX 5 (AUX Data).AUX 2_1"=w78, "MX 5 (AUX Data).AUX 2_2"=w78, "MX 5 (AUX Data).AUX 3_1"=w77, "MX 5 (AUX Data).AUX 3_2"=w77, "MX 5 (AUX Data).AUX 4_1"=w76, "MX 5 (AUX Data).AUX 4_2"=w76, "MX 5 (AUX Data).AUX 5_1"=w75, "MX 5 (AUX Data).AUX 5_2"=w75, "MX 5 (AUX Data).AUX 6_1"=w74, "MX 5 (AUX Data).AUX 6_2"=w74, "MX 5 (AUX Data).AUX 7_1"=w73, "MX 5 (AUX Data).AUX 7_2"=w73, "MX 5 (AUX Data).AUX 8_1"=w72, "MX 5 (AUX Data).AUX 8_2"=w72, "MX 5 (AUX Data).CAL CL1S"=1000.0, "MX 5 (AUX Data).CAL CL2S"=2000.0, "MX 5 (AUX Data).CAL CL3S"=3000.0, "MX 5 (AUX Data).CAL CL4S"=4000.0, "MX 5 (AUX Data).CAL CL5"=5000.0, "MX 5 (AUX Data).CAL CL6"=6000.0, "MX 5 (AUX Data).CAL CL7"=7000.0, "MX 5 (AUX Data).CAL CL8"=8000.0) -> (w80:T4)
    }
  }
  "Chamber 1 Data out" <- w11
